vi "Configure DC Source.vi"(8 "error in (no error)":errorcluster, 9 "DC Source Level (0.0 V)":dbl, 10 "DC Source State (F:Disable)":bool, 11 "VISA resource name":refnum<visa-resource-name>) -> (0 "error out":errorcluster, 3 "VISA resource name out":refnum<visa-resource-name>)   [LabVIEW 2016, in "Agilent E4980.lvlib"]
doc: "Enables or disables DC source, and setups the DC source voltage level.\n\n<B>Notes:</B>\n(1) This is valid only when your instrument installs <B>Option 001</B> (Power and DC Bias enhancement)."
uses:
  <instrlib>/Agilent E4980/Agilent E4980.lvlib
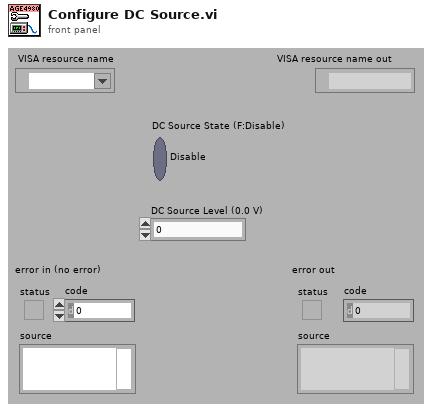
[diagram p1: front panel]
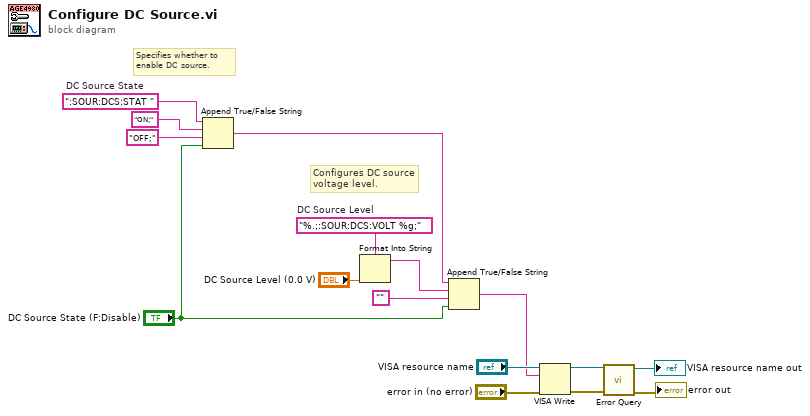
[diagram p0: block diagram]
diagram:
  w10 = "%.;:SOUR:DCS:VOLT %g;"  # DC Source Level
  w16 = ":SOUR:DCS:STAT "  # DC Source State
  # "Configures DC source\nvoltage level."
  # "Specifies whether to\nenable DC source."
  n1 = Append True/False String(1:"DC Source State (F:Disable)", 2:"OFF;" ("false string"), 3:"ON;" ("true string"), 4:w16) -> (0:w12:string)
  n2 = Format Into String(format string=w10, "DC Source Level (0.0 V)") -> (resulting string=w9:string)  [unwired: 2 in, 1 out]
  n3 = Append True/False String(1:"DC Source State (F:Disable)", 2:"" ("Empty String Constant"), 3:w9, 4:w12) -> (0:w6:string)
  n4 = VISA Write(VISA resource name="VISA resource name", write buffer=w6, error in (no error)="error in (no error)") -> (VISA resource name out=w5:refnum<visa-resource-name>, error out=w4:errorcluster)  [unwired: 1 out]
  n5 = call <instrlib>:"Error Query.vi"("error in (no error)"=w4, "VISA resource name"=w5) -> ("error out"=→"error out":errorcluster, "VISA resource name out"=→"VISA resource name out":refnum<visa-resource-name>)  [unwired: 6 in, 2 out]
